vi "OutcountHourlyByMachine.vi"(7 "Machine":string="QAMT08", 8 "error in (no error) 2":errorcluster, 9 "report in":refnum<class "NI_report.lvclass">, 10 "error in (no error)":errorcluster, 11 "connection reference":T1) -> (0 "error in (no error) 3":errorcluster, 1 "report in 2":refnum<class "NI_report.lvclass">, 2 "error out":errorcluster, 3 "connection reference 2":T1)   [LabVIEW 2012]
uses:
  <vilib>/addons/database/Connection.llb/Conn ObjectReference.ctl
  <vilib>/Utility/NIReport.llb/NI_report.lvclass
  <vilib>/addons/database/Auxilliary.llb/DB Tools Cursor Type.ctl
  <vilib>/addons/database/Connection.llb/Conn Execute.vi
  <vilib>/addons/database/Recordset.llb/Rec Fetch Recordset Data (R).vi
  <vilib>/addons/database/Recordset.llb/Rec Destroy - Connection.vi
  <vilib>/addons/database/_DB Variant To Data/Database Variant To Data.xnode
  <vilib>/Utility/NIReport.llb/Excel/NI_Excel.lvclass
  <vilib>/addons/database/NI_Database_API.lvlib
panel:
  in  "?":cluster{"start row":i32, "start column":i32}
  in  "?":cluster{"start row":i32, "start column":i32}
  in  "?":cluster{"start row":i32, "start column":i32}
  in  "?":cluster{"start row":i32, "start column":i32}
  in  "?":cluster{"start row":i32, "start column":i32}
  in  "?":cluster{"start row":i32, "start column":i32}
  in  "?":cluster{"start row":i32, "start column":i32}
  in  "?":cluster{"start row":i32, "start column":i32}
  in  "?":cluster{"start row":i32, "start column":i32}
  in  "?":cluster{"start row":i32, "start column":i32}
  in  "?":cluster{"start row":i32, "start column":i32}
  in  "?":cluster{"start row":i32, "start column":i32}
  in  "?":cluster{"start row":i32, "start column":i32}
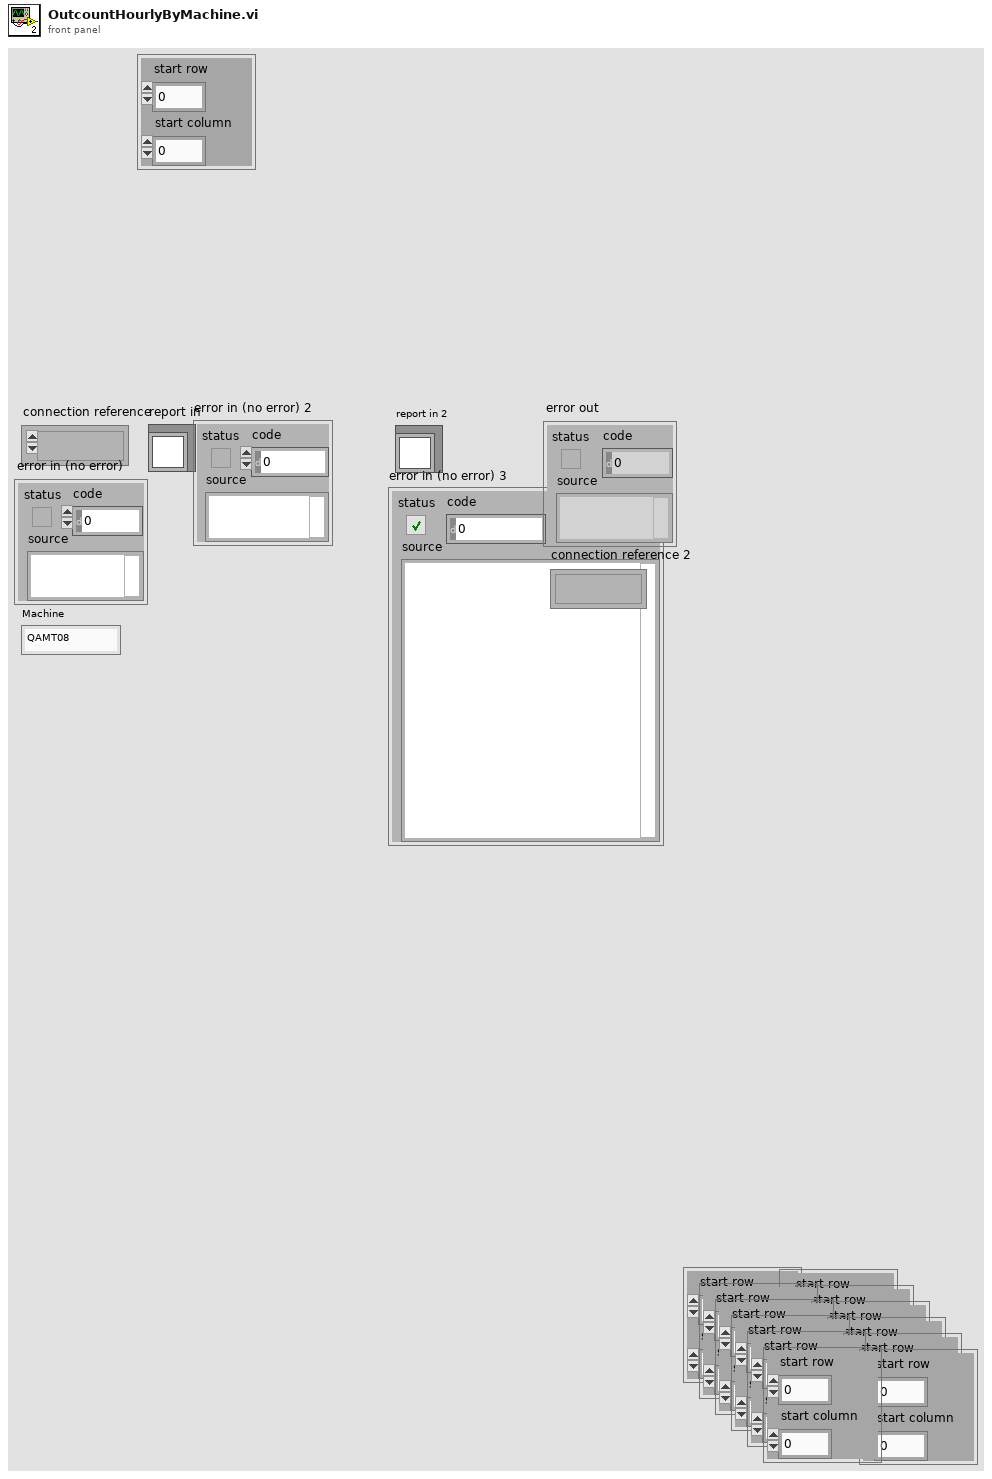
[diagram p1: front panel]
types:
  T1 = typedef "NI_Database_API.lvlib/Conn ObjectReference.ctl" = refnum<k1>
  T2 = typedef "NI_Database_API.lvlib/DB Tools Cursor Type.ctl" = enum16{"forward-only", "keyset", "dynamic", "static"}
  T3 = typedef "NI_Database_API.lvlib/Rec ObjectReference.ctl" = refnum<k1>
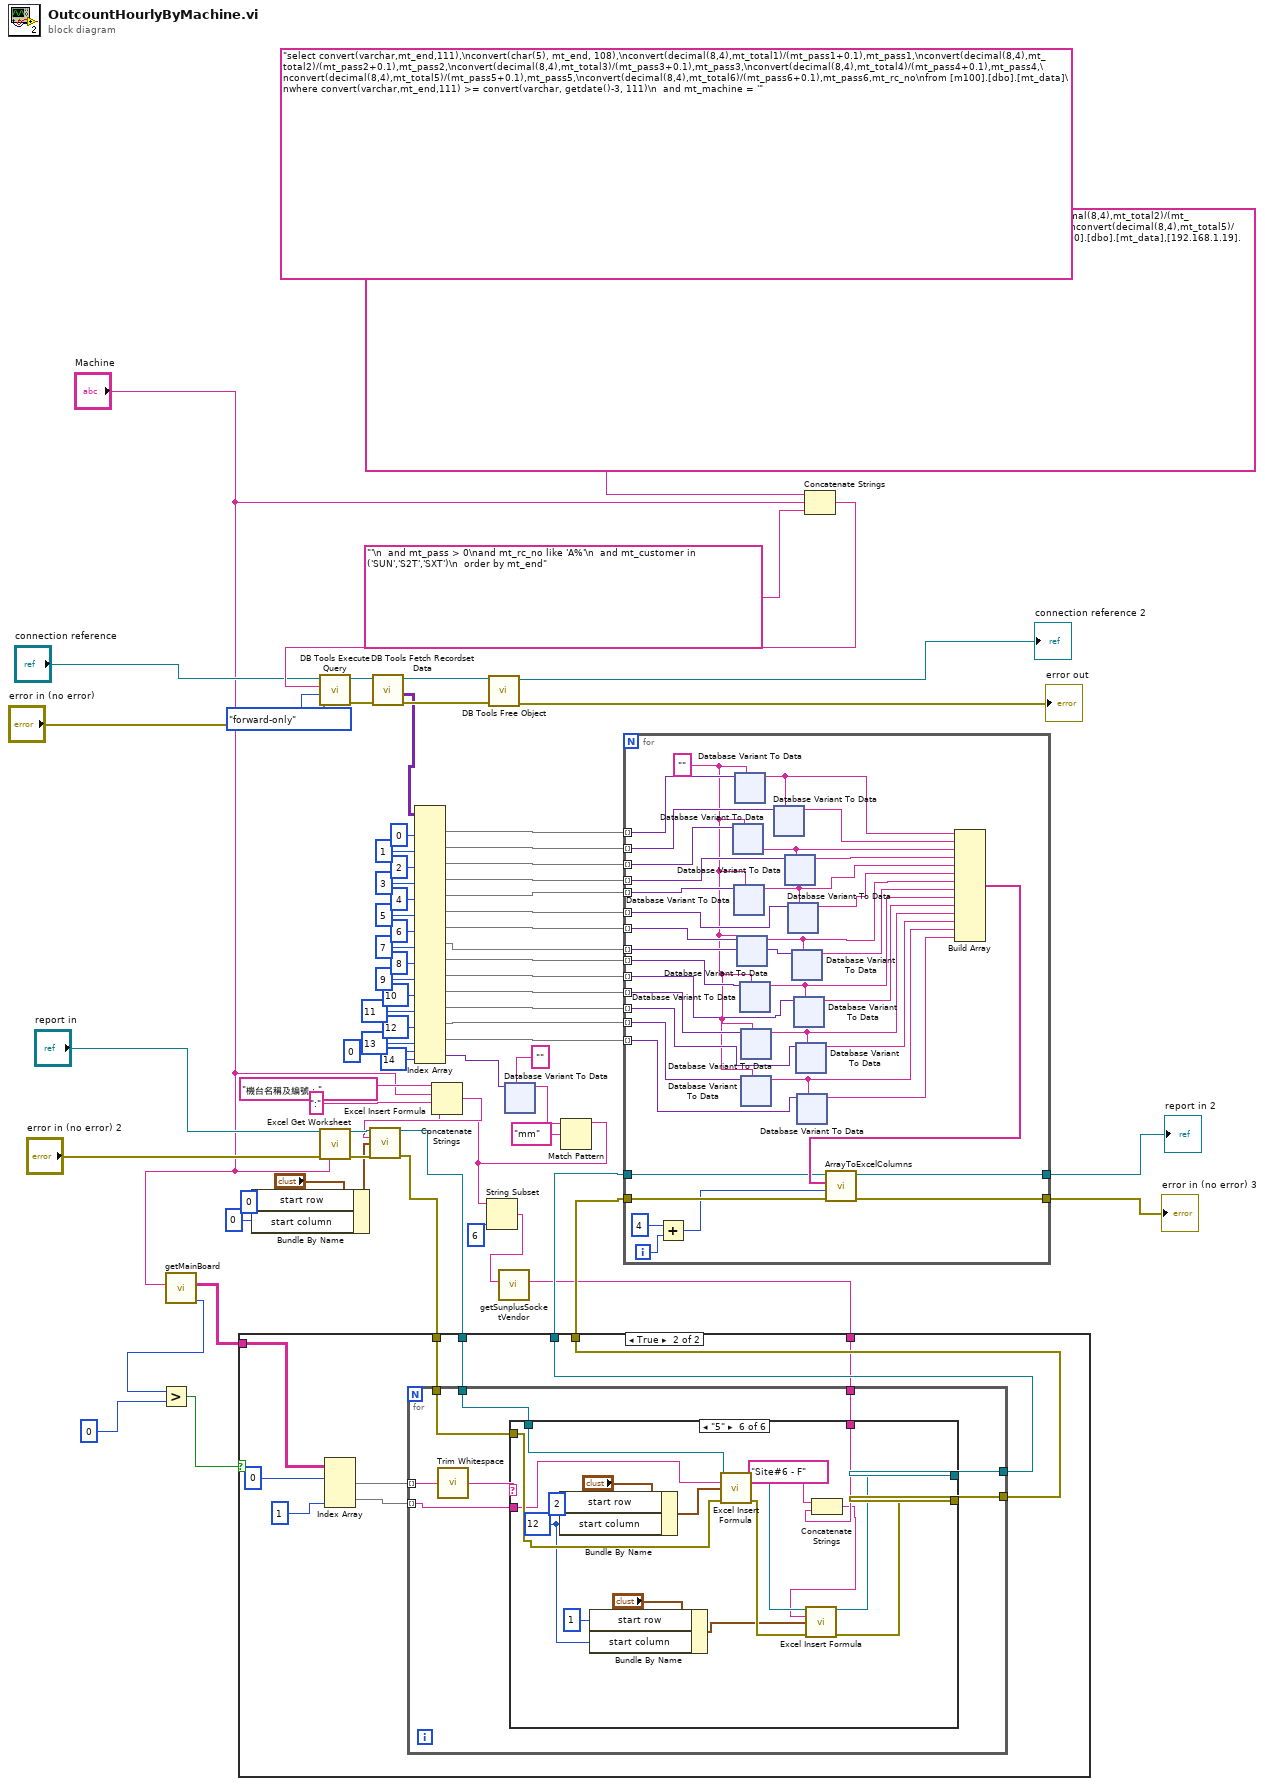
[diagram p0: block diagram]
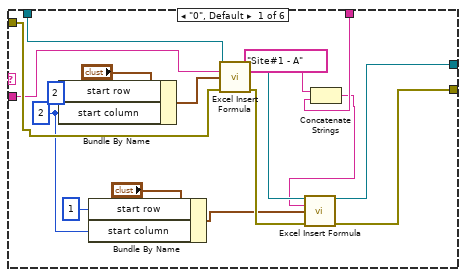
[diagram p3: hidden frame]
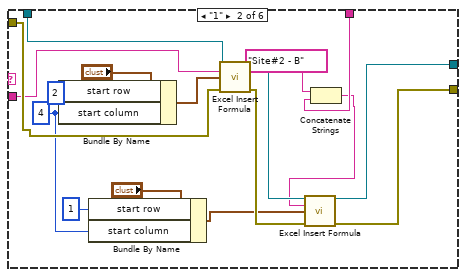
[diagram p4: hidden frame]
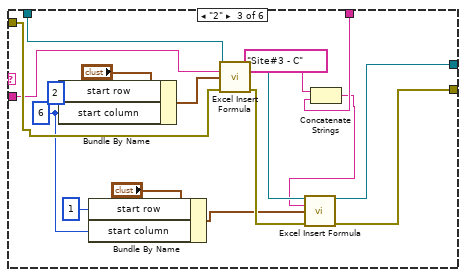
[diagram p5: hidden frame]
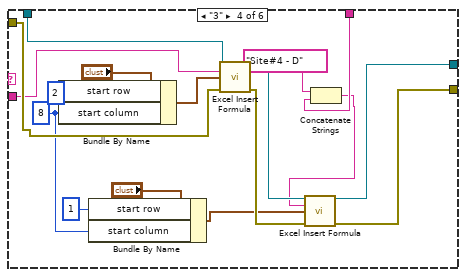
[diagram p6: hidden frame]
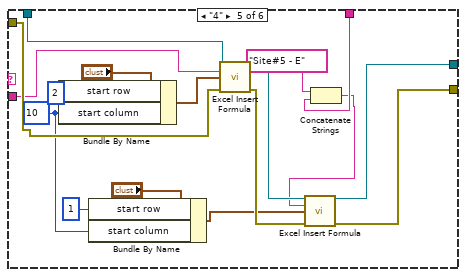
[diagram p7: hidden frame]
diagram:
  (unwired) "select convert(varchar,mt_end,111),\nconvert(char(5), mt_end, 108),\nconvert(decimal(8,4),mt_total1)/(mt_pass1+0.1),mt_pass1,\nconvert(decimal(8,4),mt_total2)/(mt_pass2+0.1),mt_pass2,\nconvert(decimal(8,4),mt_total3)/(mt_pass3+0.1),mt_pass3,\nconvert(decimal(8,4),mt_total4)/(mt_pass4+0.1),mt_pass4,\nconvert(decimal(8,4),mt_total5)/(mt_pass5+0.1),mt_pass5,\nconvert(decimal(8,4),mt_total6)/(mt_pass6+0.1),mt_pass6,mt_rc_no\nfrom [m100].[dbo].[mt_data]\nwhere convert(varchar,mt_end,111) >= convert(varchar, getdate()-3, 111)\n  and mt_machine = '" ("SQL query")
  n1 = call "getMainBoard.vi"("Machine"="Machine") -> ("Cnt"=w9:i32, "array"=w14:string[][])  [unwired: 9 in]
  n2 = Greater?(x=w9, y=0 ("Cnt")) -> (0:w7:bool)
  n3 = Bundle By Name(cluster="?", "start row"=0, "start column"=0) -> (w32:cluster{"start row":i32, "start column":i32})
  n4 = call <vilib>:"Excel Get Worksheet.vi"("report in"="report in", "error in (no error)"="error in (no error) 2", "name (\"\")"="Machine") -> ("report out"=w37:refnum<class "NI_report.lvclass">, "error out"=w36:errorcluster)  [unwired: 11 in]
  n5 = Concatenate Strings("select convert(varchar,mt_end,111),\nconvert(char(5), mt_end, 108),\nconvert(decimal(8,4),mt_total1)/(mt_pass1+0.1),mt_pass1,\nconvert(decimal(8,4),mt_total2)/(mt_pass2+0.1),mt_pass2,\nconvert(decimal(8,4),mt_total3)/(mt_pass3+0.1),mt_pass3,\nconvert(decimal(8,4),mt_total4)/(mt_pass4+0.1),mt_pass4,\nconvert(decimal(8,4),mt_total5)/(mt_pass5+0.1),mt_pass5,\nconvert(decimal(8,4),mt_total6)/(mt_pass6+0.1),mt_pass6,SUBSTRING(PRODUCTTYPE,1,6)+'_'+ BODYSIZE\nfrom [m100].[dbo].[mt_data],[192.168.1.19].[MCS].[dbo].[MCS_ASSEMBLYTYPE] ,[192.168.1.19].[MCS].[dbo].[MCS_JOB] \nwhere convert(varchar,mt_end,111) >= convert(varchar, getdate()-1, 111)\n  and ASSEMBLYTYPE=ASSEMBLYTYPENAME\n  and jobno COLLATE Chinese_Taiwan_Stroke_CI_AS = mt_rc_no\n  and mt_machine = '" ("string"), "Machine", "'\n  and mt_pass > 0\nand mt_rc_no like 'A%'\n  and mt_customer in ('SUN','S2T','SXT')\n  order by mt_end" ("SQL query")) -> (w38:string)
  n6 = call-poly <vilib>:"DB Tools Execute Query.vi"("error in (no error)"="error in (no error)", "cursor type"=DB_Tools_Cursor_Type."forward-only", "SQL query"=w38, "connection reference"="connection reference") -> ("error out"=w73:errorcluster, "recordset reference"=w72:T3)  [unwired: 4 in]
  n7 = call-poly <vilib>:"DB Tools Fetch Recordset Data.vi"("error in (no error)"=w73, "recordset reference"=w72) -> ("error out"=w70:errorcluster, "recordset data"=w68:variant[][], "recordset reference out"=w71:T3)  [unwired: 3 in]
  n8 = Index Array(array=w68, index (col) #1=0 ("disabled index (col)"), index (col) #2=1 ("index (col)"), index (col) #3=2 ("index (col)"), index (col) #4=3 ("index (col)"), index (col) #5=4 ("index (col)"), index (col) #6=5 ("index (col)"), index (col) #7=6 ("index (col)"), index (col) #8=7 ("index (col)"), index (col) #9=8 ("index (col)"), index (col) #10=9 ("index (col)"), index (col) #11=10 ("index (col)"), index (col) #12=11 ("index (col)"), index (col) #13=12 ("index (col)"), index (col) #14=13 ("index (col)"), index (row) #15=0 ("disabled index (row)"), index (col) #15=14 ("disabled index (col)")) -> (element #1=w65:variant[], element #2=w64:variant[], element #3=w63:variant[], element #4=w52:variant[], element #5=w51:variant[], element #6=w50:variant[], element #7=w49:variant[], element #8=w48:variant[], element #9=w47:variant[], element #10=w46:variant[], element #11=w45:variant[], element #12=w44:variant[], element #13=w41:variant[], element #14=w40:variant[], element #15=w18:variant)  [unwired: 14 in]
  n9 = call-poly <vilib>:"DB Tools Free Object.vi"("error in (no error)"=w70, "recordset reference"=w71) -> ("error out"=→"error out":errorcluster, "connection reference"=→"connection reference 2":T1)  [unwired: 8 in]
  n10 = xnode "Database Variant To Data"("database variant"=w18, "type"="") -> ("data"=w16:string)  [unwired: 1 in, 1 out]
  n11 = Match Pattern(string=w16, regular expression="mm") -> (before substring=w4:string)  [unwired: 1 in, 3 out]
  n12 = Concatenate Strings("機台名稱及編號：" ("formula"), "Machine", ":" ("string"), w4) -> (w31:string)
  n13 = call <vilib>:"Excel Insert Formula.vi"("report in"=w37, "formula"=w31, "start (0, 0)"=w32, "error in (no error)"=w36) -> ("report out"=w13:refnum<class "NI_report.lvclass">, "error out"=w12:errorcluster)  [unwired: 10 in]
  n14 = String Subset(string=w4, length (rest)=6 ("length (rest)")) -> (substring=w2:string)  [unwired: 1 in]
  n15 = call "getSunplusSocketVendor.vi"("Device"=w2) -> ("Vendor"=w1:string)  [unwired: 10 in]
  n16 = case shown="True" w7 {
    tunnel: w14 -> [_ w85]
    tunnel: w13 -> [w75 w81]
    tunnel: w12 -> [w74 w80]
    tunnel: [w75 w79] -> w11
    tunnel: [w74 w78] -> w10
    tunnel: w1 -> [_ w76]
    frame False {
    }
    frame True {
      n17 = Index Array(array=w85, index (col) #1=0 ("disabled index (col)"), index (col) #2=1 ("index (col)")) -> (element #1=w77:string[], element #2=w82:string[])  [unwired: 2 in]
      n18 = for {
        tunnel: w82 -> [w89] mode=indexing
        tunnel: w81 -> [w93]
        tunnel: w80 -> [w92]
        tunnel: [w91] -> w79
        tunnel: [w90] -> w78
        tunnel: w77 -> [w88] mode=indexing
        tunnel: w76 -> [w86]
        n19 = call <vilib>:"Trim Whitespace.vi"("string"=w88) -> ("trimmed string"=w87:string)  [unwired: 1 in]
        n20 = case shown="\"5\"" w87 {
          tunnel: w89 -> [w105 w122 w139 w156 w173 w190]
          tunnel: w93 -> [w107 w124 w141 w158 w175 w192]
          tunnel: w92 -> [w106 w123 w140 w157 w174 w191]
          tunnel: [w104 w121 w138 w155 w172 w189] -> w91
          tunnel: [w103 w120 w137 w154 w171 w188] -> w90
          tunnel: w86 -> [w96 w113 w130 w147 w164 w181]
          frame "0", Default {
            w99 = 2 ("start column")
            n21 = Bundle By Name(cluster="?", "start row"=2, "start column"=w99) -> (w108:cluster{"start row":i32, "start column":i32})
            n22 = Bundle By Name(cluster="?", "start row"=1, "start column"=w99) -> (w98:cluster{"start row":i32, "start column":i32})
            n23 = call <vilib>:"Excel Insert Formula.vi"("report in"=w107, "formula"=w105, "start (0, 0)"=w108, "error in (no error)"=w106) -> ("report out"=w95:refnum<class "NI_report.lvclass">, "error out"=w102:errorcluster)  [unwired: 10 in]
            n24 = Concatenate Strings("Site#1 - A" ("string"), w96) -> (w94:string)
            n25 = call <vilib>:"Excel Insert Formula.vi"("report in"=w95, "formula"=w94, "start (0, 0)"=w98, "error in (no error)"=w102) -> ("report out"=w104:refnum<class "NI_report.lvclass">, "error out"=w103:errorcluster)  [unwired: 10 in]
          }
          frame "1" {
            w116 = 4 ("start column")
            n26 = Bundle By Name(cluster="?", "start row"=2, "start column"=w116) -> (w125:cluster{"start row":i32, "start column":i32})
            n27 = Bundle By Name(cluster="?", "start row"=1, "start column"=w116) -> (w115:cluster{"start row":i32, "start column":i32})
            n28 = call <vilib>:"Excel Insert Formula.vi"("report in"=w124, "formula"=w122, "start (0, 0)"=w125, "error in (no error)"=w123) -> ("report out"=w112:refnum<class "NI_report.lvclass">, "error out"=w119:errorcluster)  [unwired: 10 in]
            n29 = Concatenate Strings("Site#2 - B" ("string"), w113) -> (w111:string)
            n30 = call <vilib>:"Excel Insert Formula.vi"("report in"=w112, "formula"=w111, "start (0, 0)"=w115, "error in (no error)"=w119) -> ("report out"=w121:refnum<class "NI_report.lvclass">, "error out"=w120:errorcluster)  [unwired: 10 in]
          }
          frame "2" {
            w133 = 6 ("start column")
            n31 = Bundle By Name(cluster="?", "start row"=2, "start column"=w133) -> (w142:cluster{"start row":i32, "start column":i32})
            n32 = Bundle By Name(cluster="?", "start row"=1, "start column"=w133) -> (w132:cluster{"start row":i32, "start column":i32})
            n33 = call <vilib>:"Excel Insert Formula.vi"("report in"=w141, "formula"=w139, "start (0, 0)"=w142, "error in (no error)"=w140) -> ("report out"=w129:refnum<class "NI_report.lvclass">, "error out"=w136:errorcluster)  [unwired: 10 in]
            n34 = Concatenate Strings("Site#3 - C" ("string"), w130) -> (w128:string)
            n35 = call <vilib>:"Excel Insert Formula.vi"("report in"=w129, "formula"=w128, "start (0, 0)"=w132, "error in (no error)"=w136) -> ("report out"=w138:refnum<class "NI_report.lvclass">, "error out"=w137:errorcluster)  [unwired: 10 in]
          }
          frame "3" {
            w150 = 8 ("start column")
            n36 = Bundle By Name(cluster="?", "start row"=2, "start column"=w150) -> (w159:cluster{"start row":i32, "start column":i32})
            n37 = Bundle By Name(cluster="?", "start row"=1, "start column"=w150) -> (w149:cluster{"start row":i32, "start column":i32})
            n38 = call <vilib>:"Excel Insert Formula.vi"("report in"=w158, "formula"=w156, "start (0, 0)"=w159, "error in (no error)"=w157) -> ("report out"=w146:refnum<class "NI_report.lvclass">, "error out"=w153:errorcluster)  [unwired: 10 in]
            n39 = Concatenate Strings("Site#4 - D" ("string"), w147) -> (w145:string)
            n40 = call <vilib>:"Excel Insert Formula.vi"("report in"=w146, "formula"=w145, "start (0, 0)"=w149, "error in (no error)"=w153) -> ("report out"=w155:refnum<class "NI_report.lvclass">, "error out"=w154:errorcluster)  [unwired: 10 in]
          }
          frame "4" {
            w167 = 10 ("start column")
            n41 = Bundle By Name(cluster="?", "start row"=2, "start column"=w167) -> (w176:cluster{"start row":i32, "start column":i32})
            n42 = Bundle By Name(cluster="?", "start row"=1, "start column"=w167) -> (w166:cluster{"start row":i32, "start column":i32})
            n43 = call <vilib>:"Excel Insert Formula.vi"("report in"=w175, "formula"=w173, "start (0, 0)"=w176, "error in (no error)"=w174) -> ("report out"=w163:refnum<class "NI_report.lvclass">, "error out"=w170:errorcluster)  [unwired: 10 in]
            n44 = Concatenate Strings("Site#5 - E" ("string"), w164) -> (w162:string)
            n45 = call <vilib>:"Excel Insert Formula.vi"("report in"=w163, "formula"=w162, "start (0, 0)"=w166, "error in (no error)"=w170) -> ("report out"=w172:refnum<class "NI_report.lvclass">, "error out"=w171:errorcluster)  [unwired: 10 in]
          }
          frame "5" {
            w184 = 12 ("start column")
            n46 = Bundle By Name(cluster="?", "start row"=2, "start column"=w184) -> (w193:cluster{"start row":i32, "start column":i32})
            n47 = Bundle By Name(cluster="?", "start row"=1, "start column"=w184) -> (w183:cluster{"start row":i32, "start column":i32})
            n48 = call <vilib>:"Excel Insert Formula.vi"("report in"=w192, "formula"=w190, "start (0, 0)"=w193, "error in (no error)"=w191) -> ("report out"=w180:refnum<class "NI_report.lvclass">, "error out"=w187:errorcluster)  [unwired: 10 in]
            n49 = Concatenate Strings("Site#6 - F" ("string"), w181) -> (w179:string)
            n50 = call <vilib>:"Excel Insert Formula.vi"("report in"=w180, "formula"=w179, "start (0, 0)"=w183, "error in (no error)"=w187) -> ("report out"=w189:refnum<class "NI_report.lvclass">, "error out"=w188:errorcluster)  [unwired: 10 in]
          }
        }
      }
    }
  }
  n51 = for {
    tunnel: w65 -> [w232] mode=indexing
    tunnel: w64 -> [w231] mode=indexing
    tunnel: w63 -> [w230] mode=indexing
    tunnel: w52 -> [w228] mode=indexing
    tunnel: w51 -> [w224] mode=indexing
    tunnel: w50 -> [w222] mode=indexing
    tunnel: w49 -> [w220] mode=indexing
    tunnel: w48 -> [w217] mode=indexing
    tunnel: w47 -> [w216] mode=indexing
    tunnel: w46 -> [w215] mode=indexing
    tunnel: w45 -> [w212] mode=indexing
    tunnel: w44 -> [w211] mode=indexing
    tunnel: w41 -> [w208] mode=indexing
    tunnel: w40 -> [w207] mode=indexing
    tunnel: w11 -> [w202]
    tunnel: w10 -> [w201]
    tunnel: [w197] -> w25
    tunnel: [w196] -> w24
    i -> [w200]
    w204 = ""
    n52 = Add(x=4, y=w200) -> (x+y=w198:i32)
    n53 = xnode "Database Variant To Data"("database variant"=w230, "type"=w204) -> ("data"=w226:string)  [unwired: 1 in, 1 out]
    n54 = xnode "Database Variant To Data"("database variant"=w224, "type"=w204) -> ("data"=w223:string)  [unwired: 1 in, 1 out]
    n55 = xnode "Database Variant To Data"("database variant"=w232, "type"=w204) -> ("data"=w227:string)  [unwired: 1 in, 1 out]
    n56 = xnode "Database Variant To Data"("database variant"=w220, "type"=w204) -> ("data"=w219:string)  [unwired: 1 in, 1 out]
    n57 = xnode "Database Variant To Data"("database variant"=w216, "type"=w204) -> ("data"=w214:string)  [unwired: 1 in, 1 out]
    n58 = xnode "Database Variant To Data"("database variant"=w212, "type"=w204) -> ("data"=w210:string)  [unwired: 1 in, 1 out]
    n59 = xnode "Database Variant To Data"("database variant"=w208, "type"=w204) -> ("data"=w206:string)  [unwired: 1 in, 1 out]
    n60 = xnode "Database Variant To Data"("database variant"=w231, "type"=w227) -> ("data"=w229:string)  [unwired: 1 in, 1 out]
    n61 = xnode "Database Variant To Data"("database variant"=w228, "type"=w226) -> ("data"=w225:string)  [unwired: 1 in, 1 out]
    n62 = xnode "Database Variant To Data"("database variant"=w222, "type"=w223) -> ("data"=w221:string)  [unwired: 1 in, 1 out]
    n63 = xnode "Database Variant To Data"("database variant"=w217, "type"=w219) -> ("data"=w218:string)  [unwired: 1 in, 1 out]
    n64 = xnode "Database Variant To Data"("database variant"=w215, "type"=w214) -> ("data"=w213:string)  [unwired: 1 in, 1 out]
    n65 = xnode "Database Variant To Data"("database variant"=w211, "type"=w210) -> ("data"=w209:string)  [unwired: 1 in, 1 out]
    n66 = xnode "Database Variant To Data"("database variant"=w207, "type"=w206) -> ("data"=w205:string)  [unwired: 1 in, 1 out]
    n67 = Build Array(w227, w229, w226, w225, w223, w221, w219, w218, w214, w213, w210, w209, w206, w205) -> (w203:string[])
    n68 = call "ArrayToExcelColumns.vi"("error in (no error)"=w201, "start row"=w198, "ArrayData"=w203, "report in"=w202) -> ("error in (no error) 2"=w196:errorcluster, "report in 2"=w197:refnum<class "NI_report.lvclass">)  [unwired: 6 in]
  }
  "report in 2" <- w25
  "error in (no error) 3" <- w24
